vi "PMR_Main.vi"() -> ()   [LabVIEW 2016, in "Budda_V2.lvrbt"]
uses:
  Budda_V2.lvrbt
  <vilib>/NXT/Block Support/NXT_InputPort.ctl
  <vilib>/NXT/Subs/ColorSensorColors.ctl
  <vilib>/NXT/Block Support/NXT_OutputPort.ctl
  <vilib>/NXT/Dual Mode Library/Sensors/EV3_Color_Color.vi
  <vilib>/NXT/Dual Mode Library/Sensors/EV3_Ultrasonic_CM.vi
  <vilib>/NXT/NXTIO Xnodes/NXTIONodeSubVIs/NXTMoveMotors.vi
  <vilib>/NXT/Dual Mode Library/Sensors/EV3_Gyro_Reset.vi
  <vilib>/NXT/Dual Mode Library/Sensors/EV3_Gyro_Angle.vi
  <vilib>/NXT/NXTIO Xnodes/NXTIONodeSubVIs/NXTStopMotors.vi
  <vilib>/NXT/Dual Mode Library/Sensors/EV3_Gyro_Rate.vi
  <vilib>/NXT/Dual Mode Library/Sound/PlayC.vi
  <vilib>/NXT/Dual Mode Library/Sound/PlayG.vi
  <vilib>/NXT/Subs/LVHSConnector.ctl
  <vilib>/NXT/NXTIO Xnodes/AddressXNode/NXTIOAddress.xnode
  <vilib>/NXT/NXTIO Xnodes/NXTIOXNode/NXTIO.xnode
  <vilib>/NXT/LegoClasses/BrickReference/BrickReference.lvclass
panel:
  in  "Nav Speed":dbl=40.0
  in  "-Grab Power":dbl=-50.0
  in  "-Turn Speed":dbl=-45.0
  out "Drop Counter":dbl
  out "Weight":string
  out "Ultrasonic Distance":dbl
  out "Current State":string
  in  "UTurn Time":dbl=2400.0
  in  "Grab Power":dbl=80.0
  in  "Weight Threshold":dbl=-20.0
  in  "Pickup Distance":dbl=7.0
  in  "Turn speed":dbl=45.0
  in  "Drive Speed":dbl=40.0
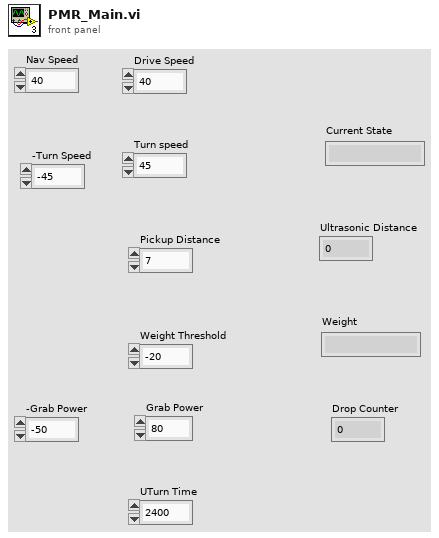
[diagram p1: front panel]
types:
  T1 = typedef "ColorSensorColors.ctl" = enum16{"No Color", "Black", "Blue", "Green", "Yellow", "Red", "White", "Brown"}
  T2 = typedef "NXT_InputPort.ctl" = u32
  T3 = typedef "NXT_OutputPort.ctl" = u8
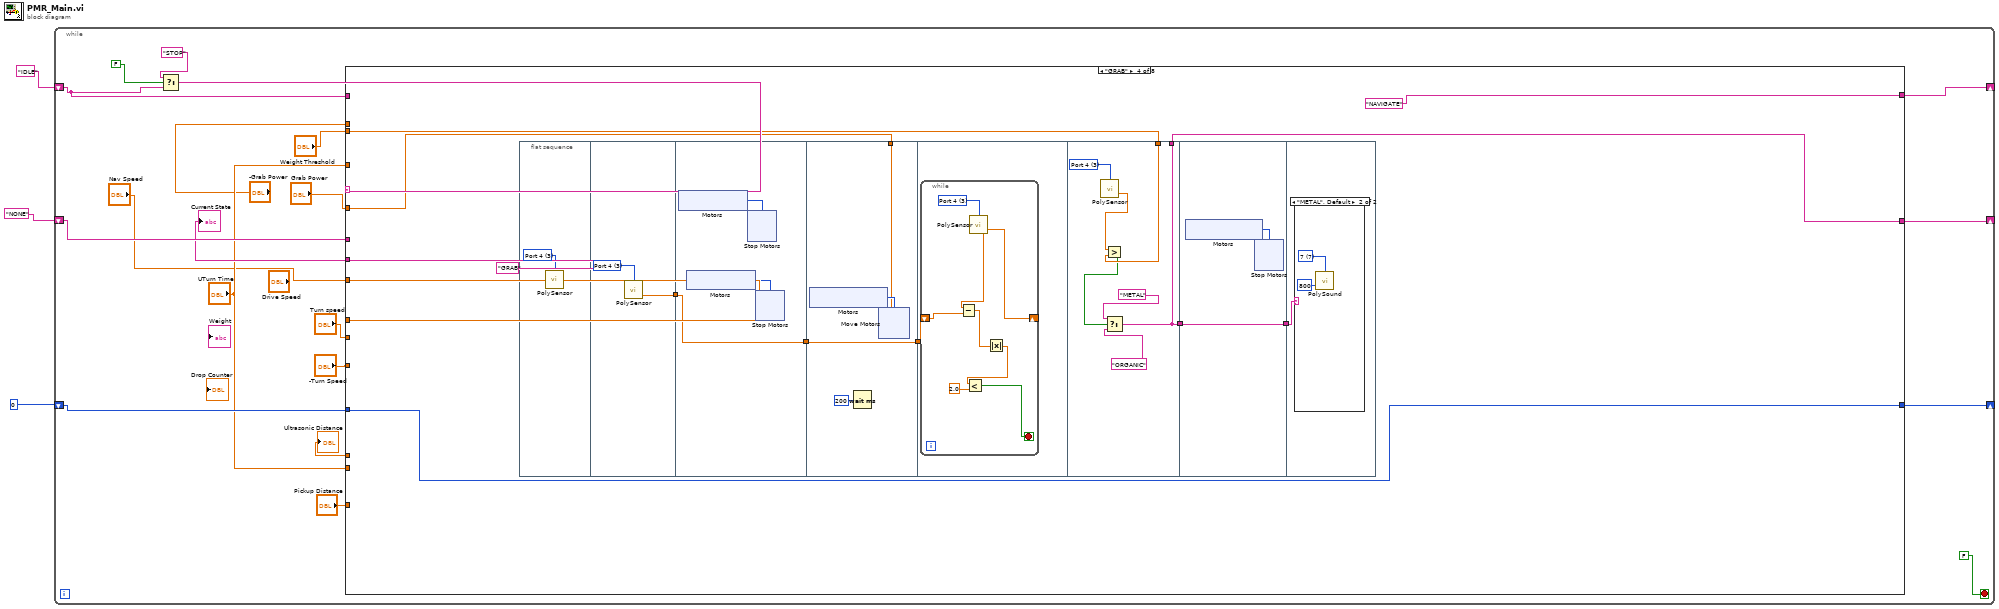
[diagram p0: block diagram]
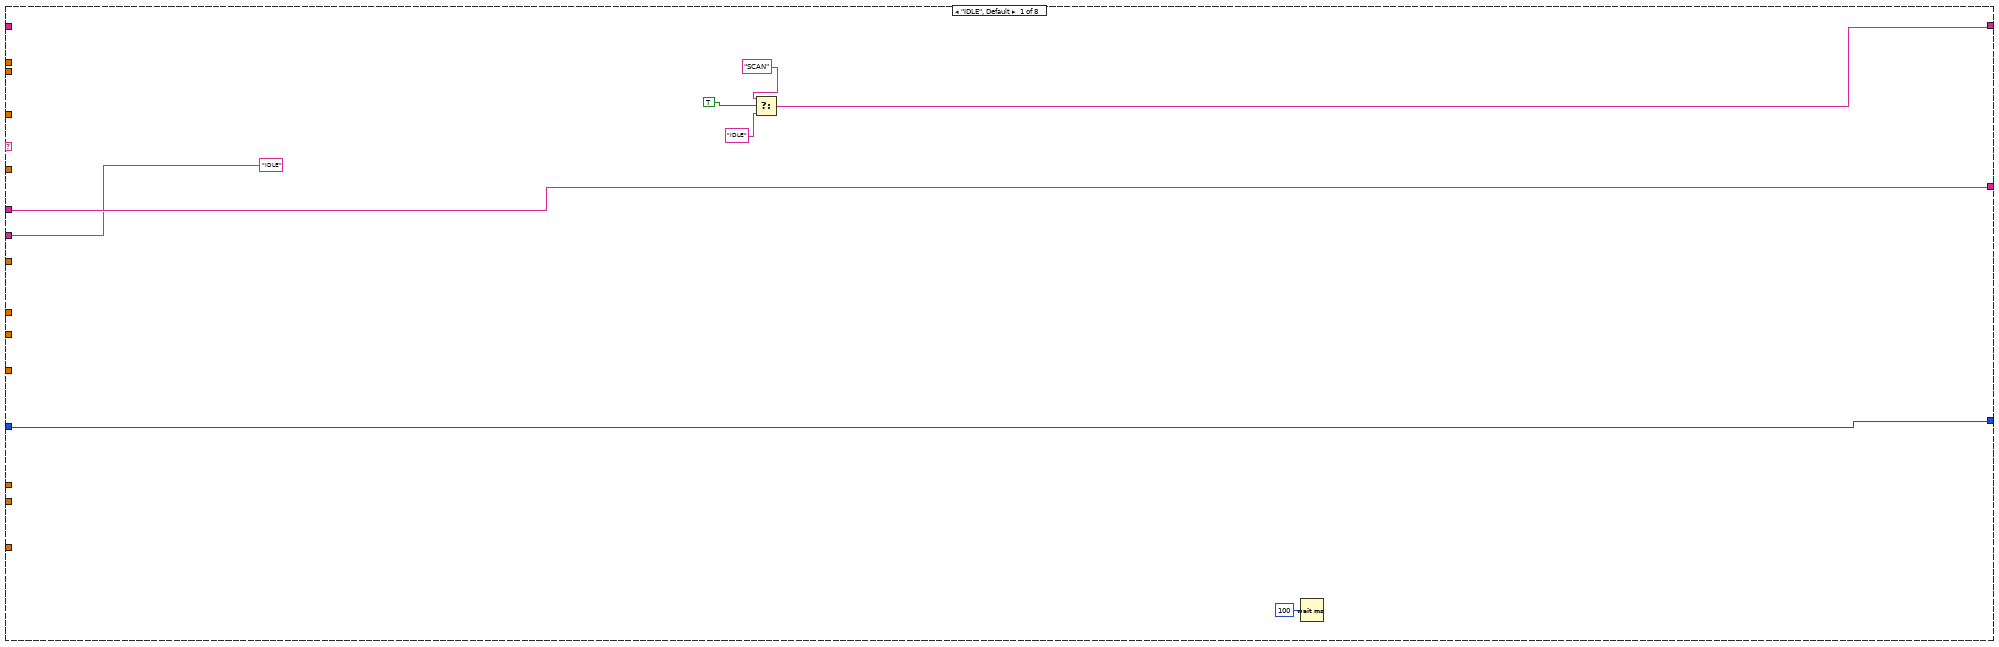
[diagram p2: hidden frame]
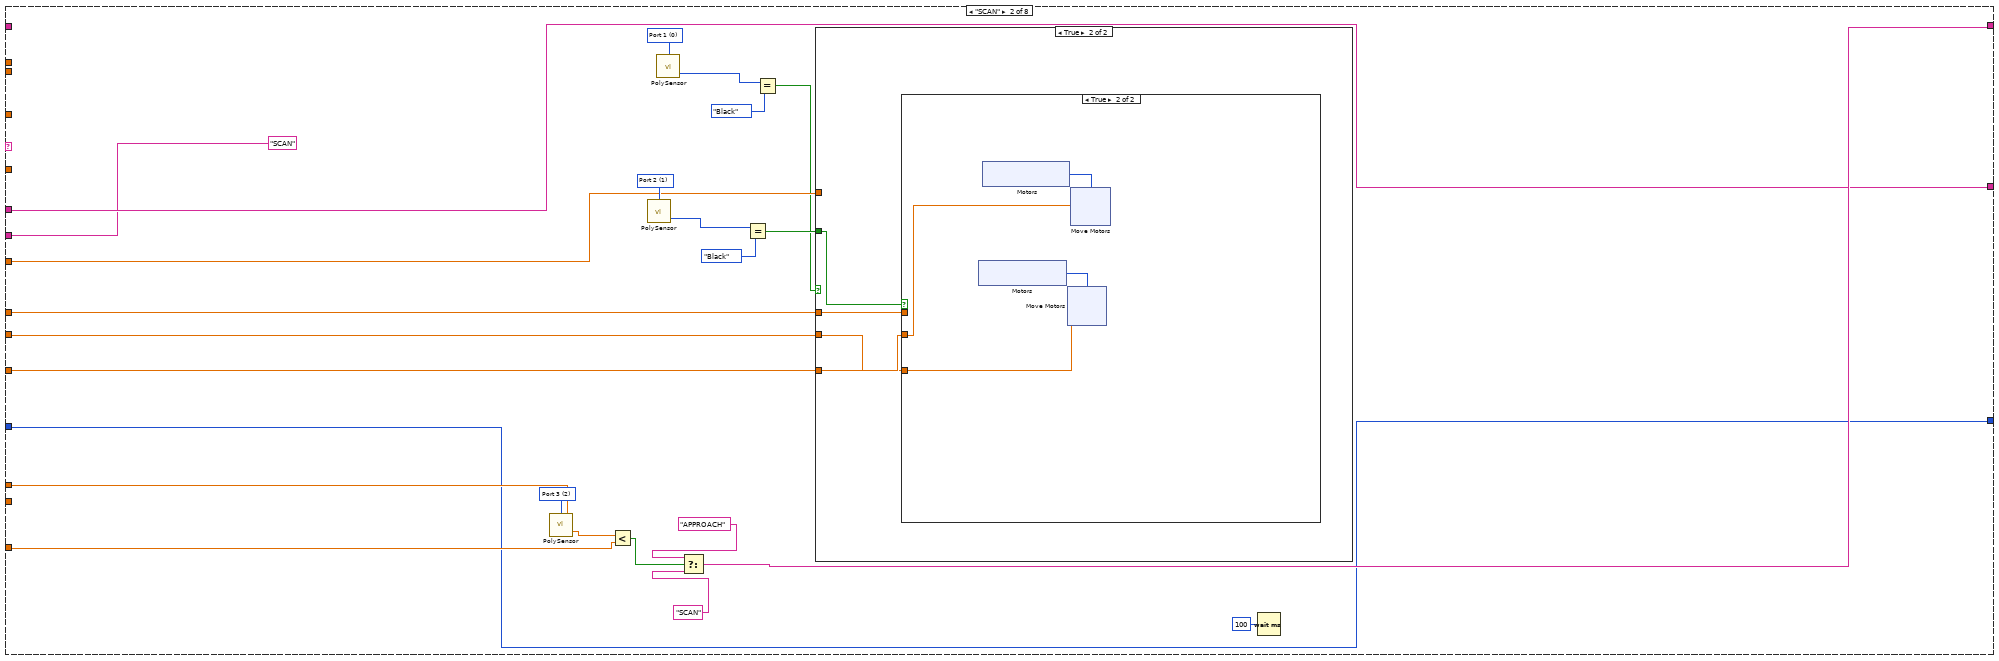
[diagram p3: hidden frame]
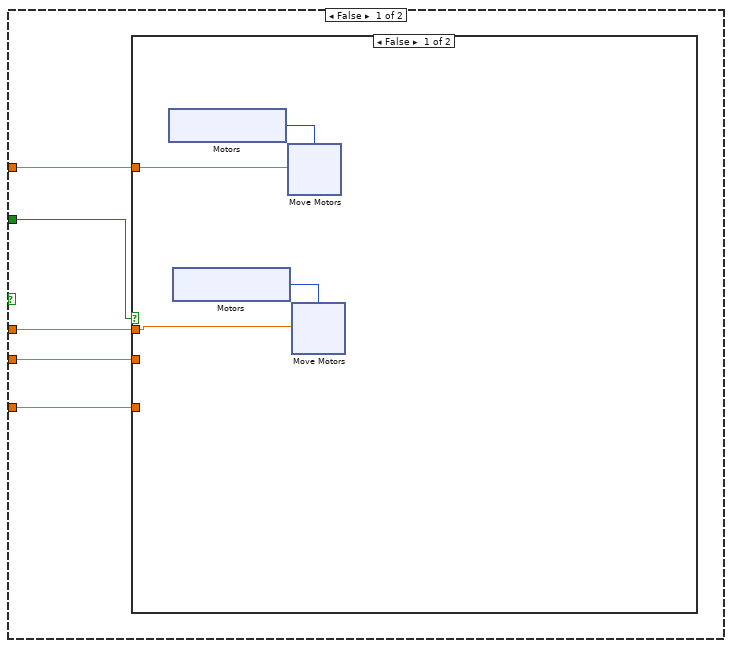
[diagram p4: hidden frame]
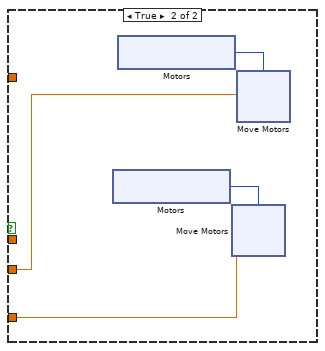
[diagram p5: hidden frame]
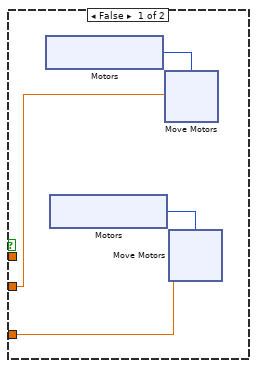
[diagram p6: hidden frame]
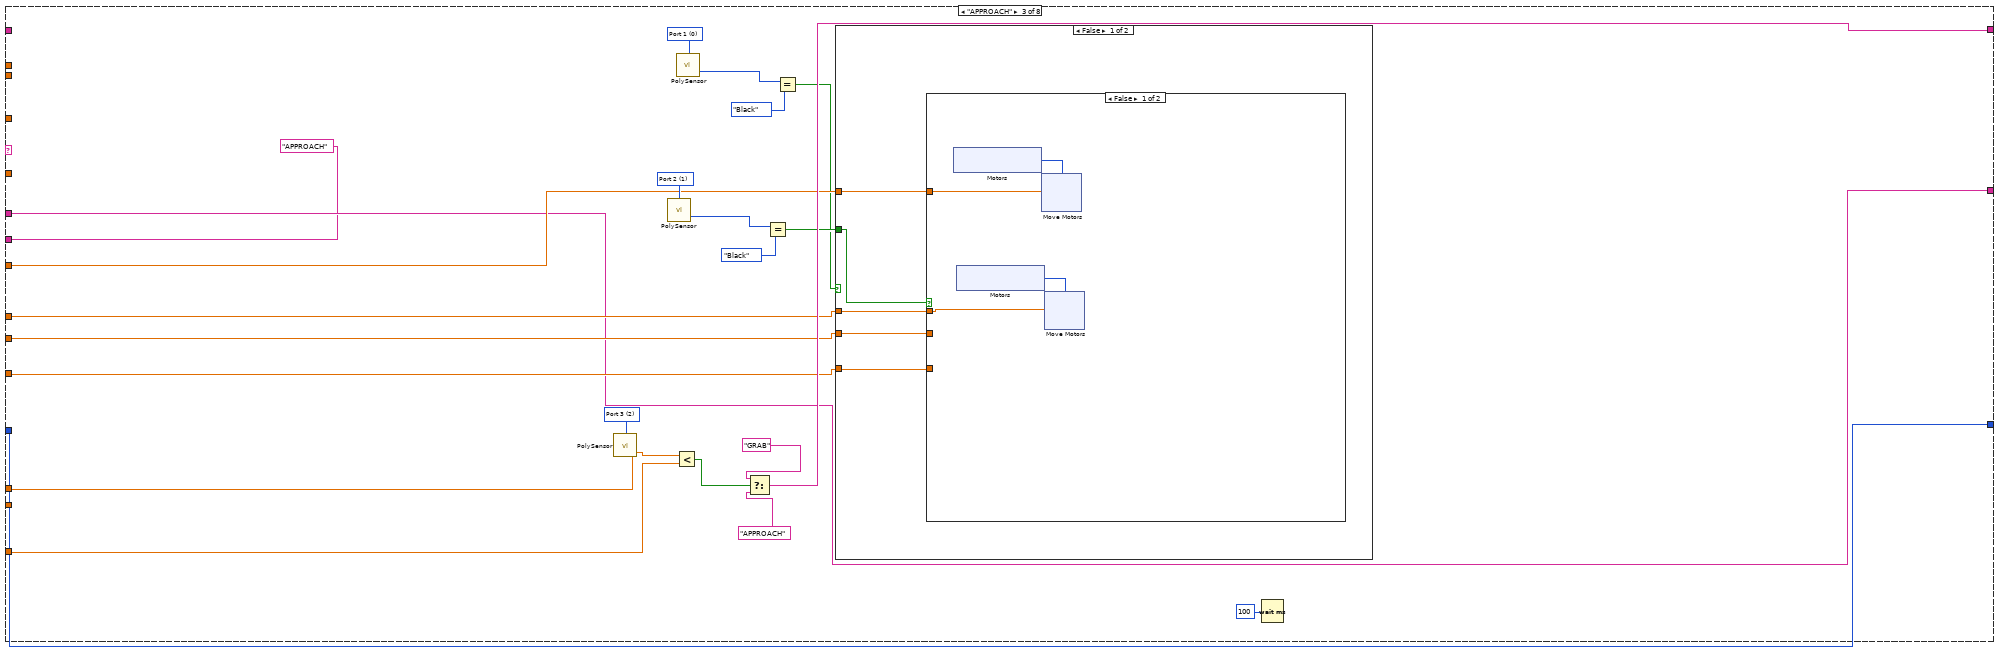
[diagram p7: hidden frame]
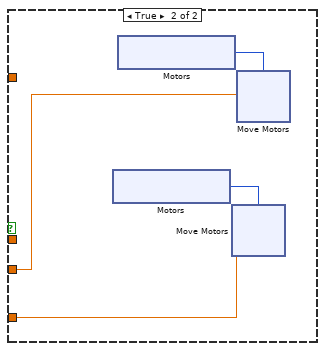
[diagram p8: hidden frame]
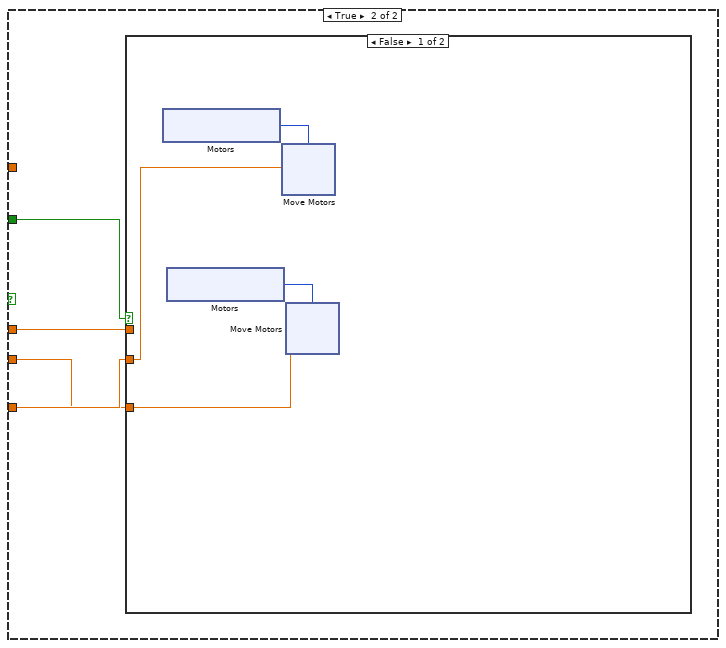
[diagram p9: hidden frame]
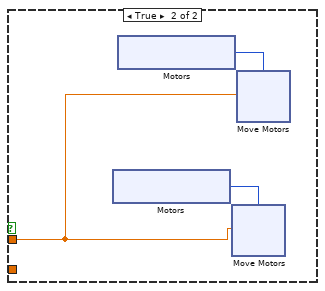
[diagram p10: hidden frame]
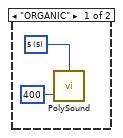
[diagram p11: hidden frame]
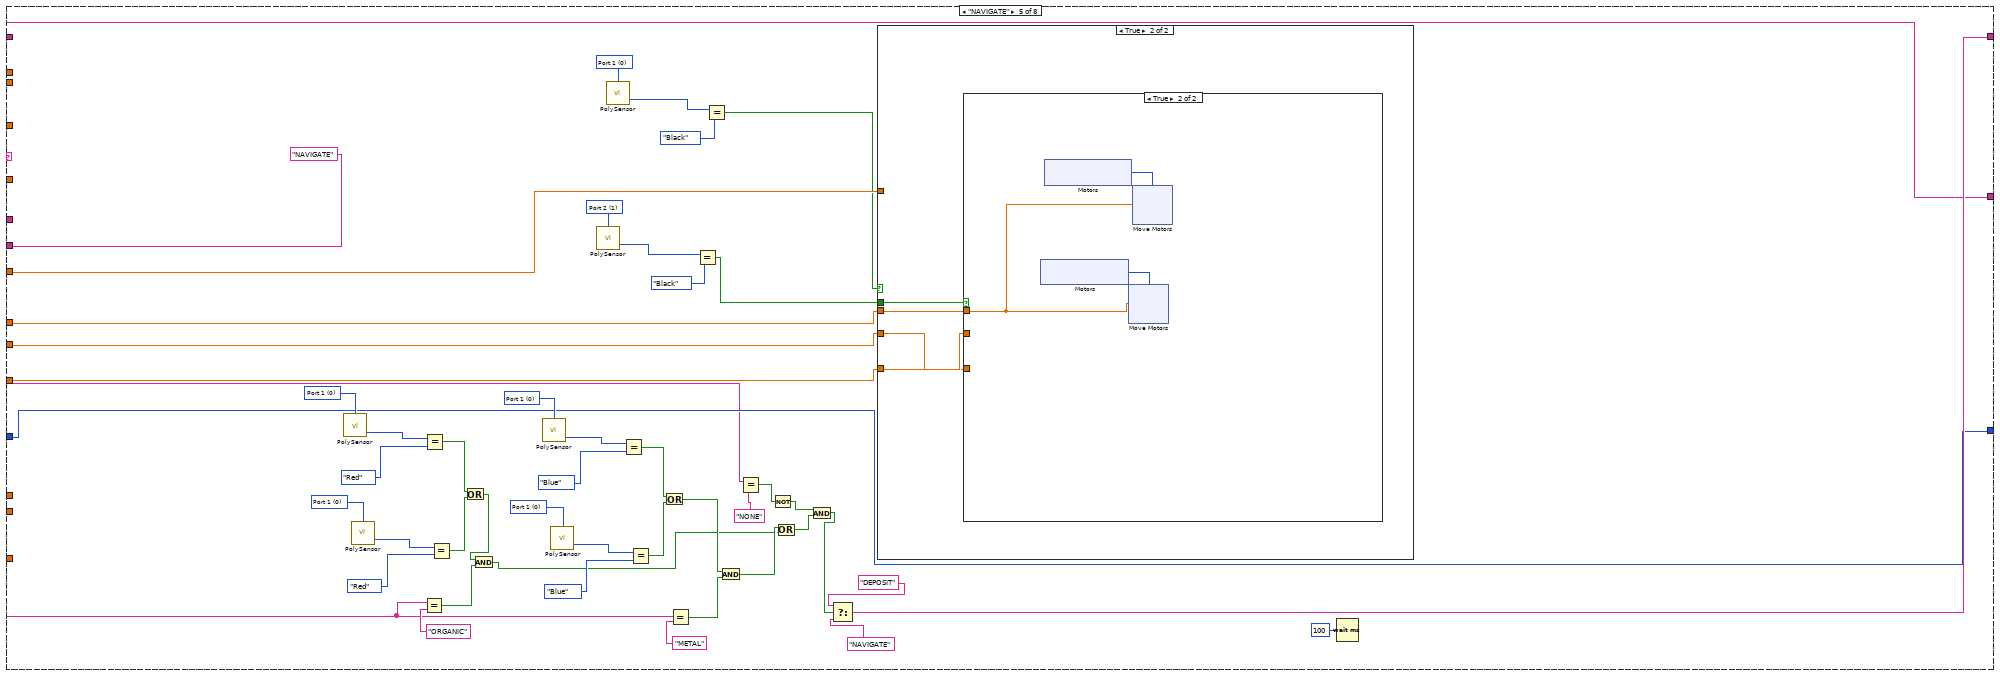
[diagram p12: hidden frame]
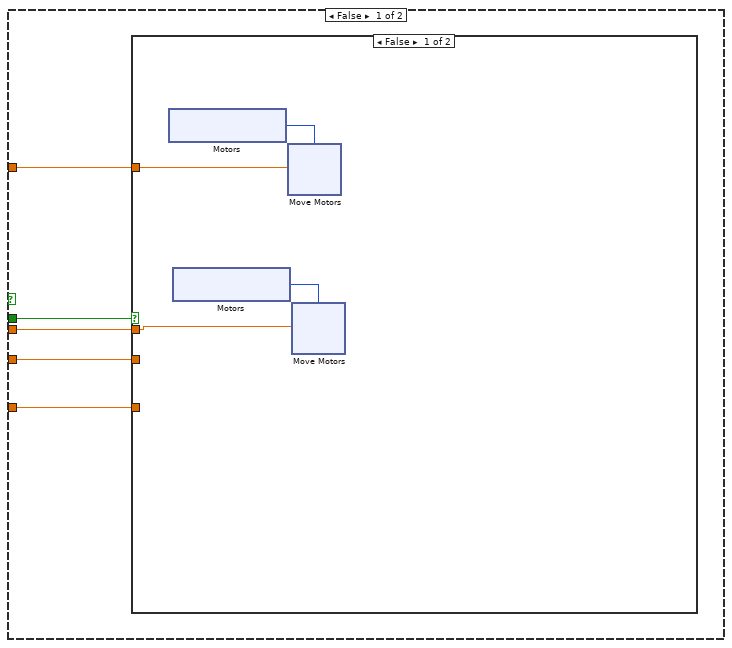
[diagram p13: hidden frame]
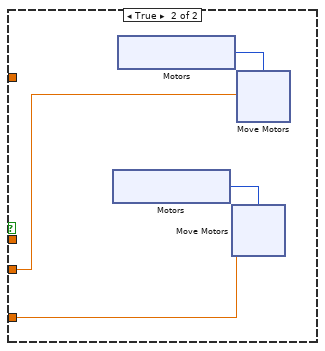
[diagram p14: hidden frame]
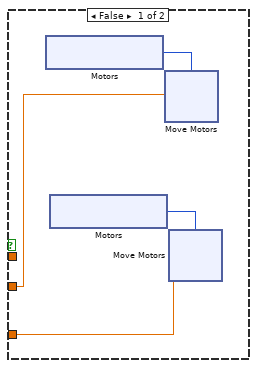
[diagram p15: hidden frame]
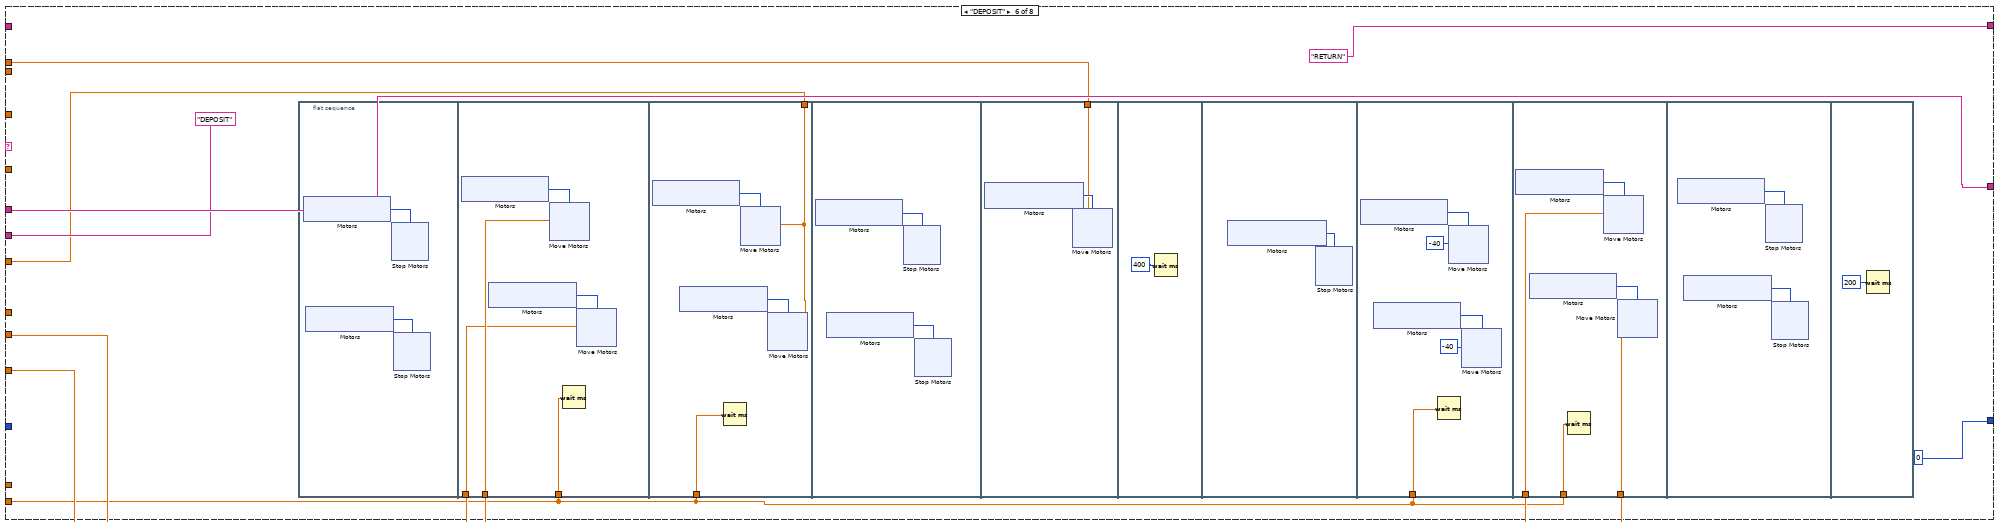
[diagram p16: hidden frame]
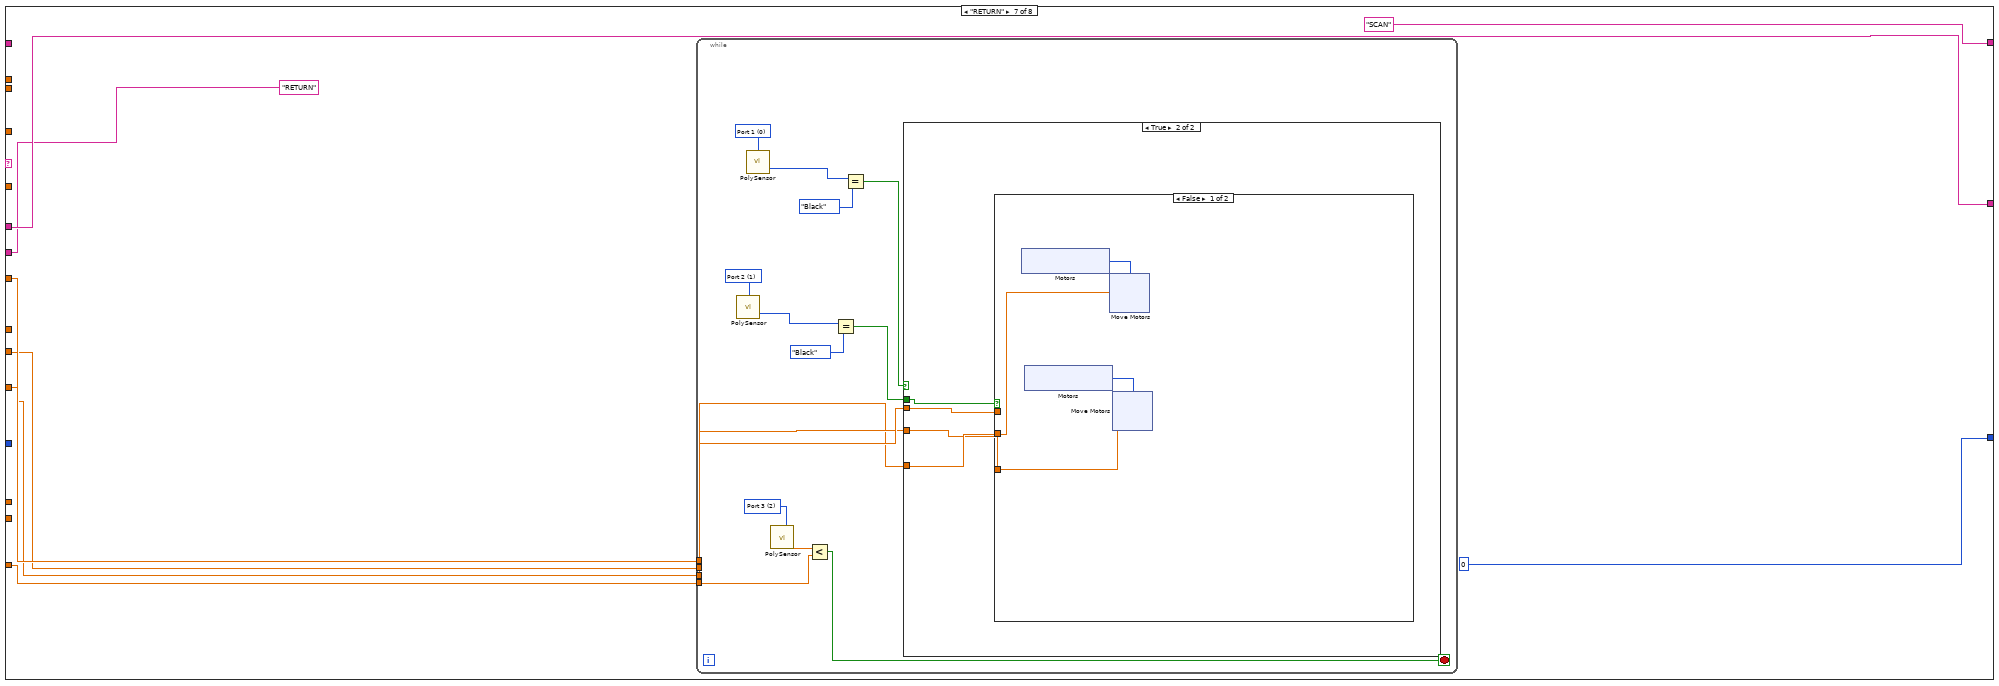
[diagram p17: hidden frame]
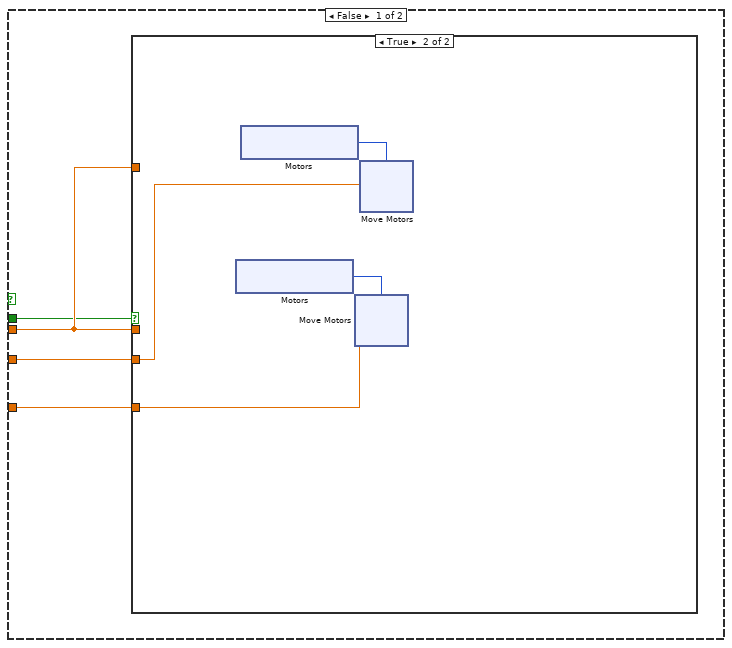
[diagram p18: hidden frame]
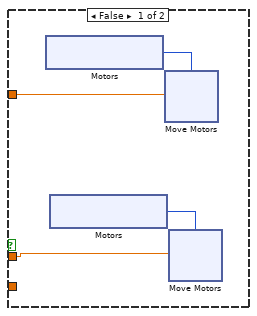
[diagram p19: hidden frame]
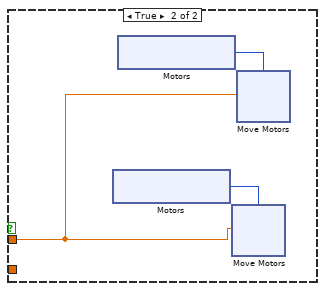
[diagram p20: hidden frame]
diagram:
  n1 = while {
    shift-right: [w11] -> _
    shift-left: "IDLE" -> [w21]
    shift-right: [w10] -> _
    shift-left: "NONE" -> [w20]
    shift-right: [w9] -> _
    shift-left: 0 -> [w19]
    stop <- FALSE stop-if-true
    n2 = Select(t="STOP", s=FALSE, f=w21) -> (s? t:f=w22:string)
    n3 = case shown="\"GRAB\"" w22 {
      tunnel: [w28 w38 w154 "NAVIGATE" w331 "RETURN" "SCAN" "IDLE"] -> w11
      tunnel: w21 -> [_ _ _ _ _ _ _ _]
      tunnel: [w26 w37 w149 w263 w327 w466 w616 w724] -> w10
      tunnel: w20 -> [w26 w37 w149 _ w327 w466 w616 w724]
      tunnel: [w31 w36 w148 w261 w330 0 0 0] -> w9
      tunnel: w19 -> [w31 w36 w148 w261 w330 _ _ _]
      tunnel: "Nav Speed" -> [_ w48 w150 _ w362 w464 w620 _]
      tunnel: "Nav Speed" -> [_ w47 w153 _ w365 _ _ _]
      tunnel: "Turn speed" -> [_ w46 w152 _ w364 w462 w613 _]
      tunnel: "-Turn Speed" -> [_ w45 w151 _ w363 w461 w614 _]
      tunnel: [_ w43 w155 _ _ _ _ _] -> w16
      tunnel: "Pickup Distance" -> [_ w42 w156 _ _ _ w619 _]
      tunnel: "Grab Power" -> [_ _ _ w265 _ _ _ _]
      tunnel: "Weight Threshold" -> [_ _ _ w264 _ _ _ _]
      tunnel: ["IDLE" "SCAN" "APPROACH" "GRAB" "NAVIGATE" "DEPOSIT" "RETURN" "STOP"] -> w12
      tunnel: "UTurn Time" -> [_ _ _ _ _ _ _ _]
      tunnel: "UTurn Time" -> [_ _ _ _ _ w460 _ _]
      tunnel: "-Grab Power" -> [_ _ _ _ _ w463 _ _]
      frame "IDLE", Default {
        n4 = Select(t="SCAN", s=TRUE, f="IDLE") -> (s? t:f=w28:string)
        n5 = Wait (ms)(milliseconds to wait=u32 100) -> ()  [unwired: 1 out]
      }
      frame "SCAN" {
        w44 = T2 2 items=["Port 1", "Port 2", "Port 3", "Port 4"] ("Port (Port 1)")
        w51 = T2 1 items=["Port 1", "Port 2", "Port 3", "Port 4"] ("Port (Port 1)")
        w54 = T2 0 items=["Port 1", "Port 2", "Port 3", "Port 4"] ("Port (Port 1)")
        n6 = call-poly <vilib>:"PolySensor.vi"("Port (Port 1)"=w44) -> ("Centimeters"=w43:sgl)  [unwired: 2 in, 1 out]
        n7 = Less?(x=w43, y=w42) -> (x < y?=w41:bool)
        n8 = call-poly <vilib>:"PolySensor.vi"("Port (Port 1)"=w51) -> ("Detected Color"=w50:T1)  [unwired: 2 in, 1 out]
        n9 = call-poly <vilib>:"PolySensor.vi"("Port (Port 1)"=w54) -> ("Detected Color"=w53:T1)  [unwired: 2 in, 1 out]
        n10 = Select(t="APPROACH", s=w41, f="SCAN") -> (s? t:f=w38:string)
        n11 = Equal?(x=w50, y=ColorSensorColors."Black") -> (x = y?=w33:bool)
        n12 = Equal?(x=w53, y=ColorSensorColors."Black") -> (x = y?=w32:bool)
        n13 = case shown="True" w32 {
          tunnel: w48 -> [w59 _]
          tunnel: w47 -> [w58 w101]
          tunnel: w46 -> [w57 w102]
          tunnel: w45 -> [w56 w103]
          tunnel: w33 -> [w55 w100]
          frame False {
            n14 = case shown="False" w55 {
              tunnel: w59 -> [w61 _]
              tunnel: w58 -> [w60 _]
              tunnel: w57 -> [_ w81]
              tunnel: w56 -> [_ w80]
              frame False {
                n15 = xnode "Motors"() -> ("Motor"=w63:T3)
                n16 = xnode "Motors"() -> ("Motor"=w62:T3)
                n17 = xnode "Move Motors"("Power/Speed 1"=w61, "Motors"=w63) -> ()  [unwired: 1 in, 1 out]
                n18 = xnode "Move Motors"("Power/Speed 1"=w60, "Motors"=w62) -> ()  [unwired: 1 in, 1 out]
              }
              frame True {
                n19 = xnode "Motors"() -> ("Motor"=w82:T3)
                n20 = xnode "Motors"() -> ("Motor"=w83:T3)
                n21 = xnode "Move Motors"("Power/Speed 1"=w80, "Motors"=w82) -> ()  [unwired: 1 in, 1 out]
                n22 = xnode "Move Motors"("Power/Speed 1"=w81, "Motors"=w83) -> ()  [unwired: 1 in, 1 out]
              }
            }
          }
          frame True {
            n23 = case shown="True" w100 {
              tunnel: w103 -> [w105 w125]
              tunnel: w102 -> [w104 w124]
              tunnel: w101 -> [_ _]
              frame False {
                n24 = xnode "Motors"() -> ("Motor"=w107:T3)
                n25 = xnode "Motors"() -> ("Motor"=w106:T3)
                n26 = xnode "Move Motors"("Power/Speed 1"=w105, "Motors"=w107) -> ()  [unwired: 1 in, 1 out]
                n27 = xnode "Move Motors"("Power/Speed 1"=w104, "Motors"=w106) -> ()  [unwired: 1 in, 1 out]
              }
              frame True {
                n28 = xnode "Motors"() -> ("Motor"=w126:T3)
                n29 = xnode "Motors"() -> ("Motor"=w127:T3)
                n30 = xnode "Move Motors"("Power/Speed 1"=w124, "Motors"=w126) -> ()  [unwired: 1 in, 1 out]
                n31 = xnode "Move Motors"("Power/Speed 1"=w125, "Motors"=w127) -> ()  [unwired: 1 in, 1 out]
              }
            }
          }
        }
        n32 = Wait (ms)(milliseconds to wait=u32 100) -> ()  [unwired: 1 out]
      }
      frame "APPROACH" {
        w160 = T2 2 items=["Port 1", "Port 2", "Port 3", "Port 4"] ("Port (Port 1)")
        w163 = T2 1 items=["Port 1", "Port 2", "Port 3", "Port 4"] ("Port (Port 1)")
        w166 = T2 0 items=["Port 1", "Port 2", "Port 3", "Port 4"] ("Port (Port 1)")
        n33 = call-poly <vilib>:"PolySensor.vi"("Port (Port 1)"=w160) -> ("Centimeters"=w155:sgl)  [unwired: 2 in, 1 out]
        n34 = call-poly <vilib>:"PolySensor.vi"("Port (Port 1)"=w163) -> ("Detected Color"=w162:T1)  [unwired: 2 in, 1 out]
        n35 = Less?(x=w155, y=w156) -> (x < y?=w159:bool)
        n36 = call-poly <vilib>:"PolySensor.vi"("Port (Port 1)"=w166) -> ("Detected Color"=w165:T1)  [unwired: 2 in, 1 out]
        n37 = Select(t="GRAB", s=w159, f="APPROACH") -> (s? t:f=w154:string)
        n38 = Equal?(x=w162, y=ColorSensorColors."Black") -> (x = y?=w145:bool)
        n39 = Equal?(x=w165, y=ColorSensorColors."Black") -> (x = y?=w144:bool)
        n40 = case shown="False" w144 {
          tunnel: w150 -> [w171 _]
          tunnel: w153 -> [w170 w213]
          tunnel: w152 -> [w169 w214]
          tunnel: w151 -> [w168 w215]
          tunnel: w145 -> [w167 w212]
          frame False {
            n41 = case shown="False" w167 {
              tunnel: w171 -> [w173 _]
              tunnel: w170 -> [w172 _]
              tunnel: w169 -> [_ w193]
              tunnel: w168 -> [_ w192]
              frame False {
                n42 = xnode "Motors"() -> ("Motor"=w175:T3)
                n43 = xnode "Motors"() -> ("Motor"=w174:T3)
                n44 = xnode "Move Motors"("Power/Speed 1"=w173, "Motors"=w175) -> ()  [unwired: 1 in, 1 out]
                n45 = xnode "Move Motors"("Power/Speed 1"=w172, "Motors"=w174) -> ()  [unwired: 1 in, 1 out]
              }
              frame True {
                n46 = xnode "Motors"() -> ("Motor"=w194:T3)
                n47 = xnode "Motors"() -> ("Motor"=w195:T3)
                n48 = xnode "Move Motors"("Power/Speed 1"=w192, "Motors"=w194) -> ()  [unwired: 1 in, 1 out]
                n49 = xnode "Move Motors"("Power/Speed 1"=w193, "Motors"=w195) -> ()  [unwired: 1 in, 1 out]
              }
            }
          }
          frame True {
            n50 = case shown="False" w212 {
              tunnel: w215 -> [w217 _]
              tunnel: w214 -> [w216 _]
              tunnel: w213 -> [_ w236]
              frame False {
                n51 = xnode "Motors"() -> ("Motor"=w219:T3)
                n52 = xnode "Motors"() -> ("Motor"=w218:T3)
                n53 = xnode "Move Motors"("Power/Speed 1"=w217, "Motors"=w219) -> ()  [unwired: 1 in, 1 out]
                n54 = xnode "Move Motors"("Power/Speed 1"=w216, "Motors"=w218) -> ()  [unwired: 1 in, 1 out]
              }
              frame True {
                n55 = xnode "Motors"() -> ("Motor"=w237:T3)
                n56 = xnode "Motors"() -> ("Motor"=w238:T3)
                n57 = xnode "Move Motors"("Power/Speed 1"=w236, "Motors"=w237) -> ()  [unwired: 1 in, 1 out]
                n58 = xnode "Move Motors"("Power/Speed 1"=w236, "Motors"=w238) -> ()  [unwired: 1 in, 1 out]
              }
            }
          }
        }
        n59 = Wait (ms)(milliseconds to wait=u32 100) -> ()  [unwired: 1 out]
      }
      frame "GRAB" {
        n60 = flat-sequence {
          tunnel: [w267] -> w257
          tunnel: w257 -> [w269]
          tunnel: [w269] -> w255
          tunnel: w265 -> [w286]
          tunnel: [w285] -> w256
          tunnel: w255 -> [w285]
          tunnel: w256 -> [w296]
          tunnel: w264 -> [w305]
          tunnel: [w308] -> w263
          tunnel: [w308] -> w258
          tunnel: [w311] -> w259
          tunnel: w258 -> [w311]
          tunnel: w259 -> [w319]
          frame #0 {
            w266 = T2 3 items=["Port 1", "Port 2", "Port 3", "Port 4"] ("Port (Port 1)")
            n61 = call-poly <vilib>:"PolySensor.vi"("Port (Port 1)"=w266) -> ()  [unwired: 3 in, 1 out]
          }
          frame #1 {
            w268 = T2 3 items=["Port 1", "Port 2", "Port 3", "Port 4"] ("Port (Port 1)")
            n62 = call-poly <vilib>:"PolySensor.vi"("Port (Port 1)"=w268) -> ("Degrees"=w267:sgl)  [unwired: 2 in, 1 out]
          }
          frame #2 {
            n63 = xnode "Motors"() -> ("Motor"=w271:T3)
            n64 = xnode "Motors"() -> ("Motor"=w270:T3)
            n65 = xnode "Stop Motors"("Motors"=w271) -> ()  [unwired: 1 in, 1 out]
            n66 = xnode "Stop Motors"("Motors"=w270) -> ()  [unwired: 1 in, 1 out]
          }
          frame #3 {
            n67 = xnode "Motors"() -> ("Motor"=w287:T3)
            n68 = Wait (ms)(milliseconds to wait=u32 200) -> ()  [unwired: 1 out]
            n69 = xnode "Move Motors"("Power/Speed 1"=w286, "Motors"=w287) -> ()  [unwired: 1 in, 1 out]
          }
          frame #4 {
            n70 = while {
              shift-right: [w297] -> _
              shift-left: w296 -> [w298]
              stop <- w299 stop-if-true
              w303 = T2 3 items=["Port 1", "Port 2", "Port 3", "Port 4"] ("Port (Port 1)")
              n71 = call-poly <vilib>:"PolySensor.vi"("Port (Port 1)"=w303) -> ("Degrees"=w297:sgl)  [unwired: 2 in, 1 out]
              n72 = Subtract(x=w297, y=w298) -> (x-y=w302:sgl)
              n73 = Absolute Value(x=w302) -> (abs(x)=w301:sgl)
              n74 = Less?(x=w301, y=sgl 2.0) -> (x < y?=w299:bool)
            }
          }
          frame #5 {
            w307 = T2 3 items=["Port 1", "Port 2", "Port 3", "Port 4"] ("Port (Port 1)")
            n75 = call-poly <vilib>:"PolySensor.vi"("Port (Port 1)"=w307) -> ("Degrees/Second"=w306:sgl)  [unwired: 2 in, 1 out]
            n76 = Greater?(x=w306, y=w305) -> (0:w304:bool)
            n77 = Select(t="METAL", s=w304, f="ORGANIC") -> (s? t:f=w308:string)
          }
          frame #6 {
            n78 = xnode "Motors"() -> ("Motor"=w312:T3)
            n79 = xnode "Stop Motors"("Motors"=w312) -> ()  [unwired: 1 in, 1 out]
          }
          frame #7 {
            n80 = case shown="\"METAL\", Default" w319 {
              frame "ORGANIC" {
                w320 = u16 5 items=["3"=3, "4"=4, "5"=5, "6"=6, "7"=7] ("Octave")
                n81 = call-poly <vilib>:"PolySound.vi"("Duration (500 ms)"=u16 400, "Octave"=w320) -> ()  [unwired: 2 in, 1 out]
              }
              frame "METAL", Default {
                w322 = u16 7 items=["3"=3, "4"=4, "5"=5, "6"=6, "7"=7] ("Octave")
                n82 = call-poly <vilib>:"PolySound.vi"("Duration (500 ms)"=u16 800, "Octave"=w322) -> ()  [unwired: 2 in, 1 out]
              }
            }
          }
        }
      }
      frame "NAVIGATE" {
        w346 = T2 0 items=["Port 1", "Port 2", "Port 3", "Port 4"] ("Port (Port 1)")
        w349 = T2 0 items=["Port 1", "Port 2", "Port 3", "Port 4"] ("Port (Port 1)")
        w354 = T2 0 items=["Port 1", "Port 2", "Port 3", "Port 4"] ("Port (Port 1)")
        w357 = T2 0 items=["Port 1", "Port 2", "Port 3", "Port 4"] ("Port (Port 1)")
        w368 = T2 1 items=["Port 1", "Port 2", "Port 3", "Port 4"] ("Port (Port 1)")
        w371 = T2 0 items=["Port 1", "Port 2", "Port 3", "Port 4"] ("Port (Port 1)")
        n83 = call-poly <vilib>:"PolySensor.vi"("Port (Port 1)"=w357) -> ("Detected Color"=w356:T1)  [unwired: 2 in, 1 out]
        n84 = call-poly <vilib>:"PolySensor.vi"("Port (Port 1)"=w354) -> ("Detected Color"=w353:T1)  [unwired: 2 in, 1 out]
        n85 = Equal?(x=w327, y="ORGANIC") -> (x = y?=w337:bool)
        n86 = Equal?(x=w356, y=ColorSensorColors."Red" ("Detected Color")) -> (x = y?=w351:bool)
        n87 = Equal?(x=w353, y=ColorSensorColors."Red" ("Detected Color")) -> (x = y?=w350:bool)
        n88 = Or(x=w351, y=w350) -> (x .or. y?=w336:bool)
        n89 = And(x=w336, y=w337) -> (x .and. y?=w334:bool)
        n90 = call-poly <vilib>:"PolySensor.vi"("Port (Port 1)"=w349) -> ("Detected Color"=w348:T1)  [unwired: 2 in, 1 out]
        n91 = call-poly <vilib>:"PolySensor.vi"("Port (Port 1)"=w346) -> ("Detected Color"=w345:T1)  [unwired: 2 in, 1 out]
        n92 = call-poly <vilib>:"PolySensor.vi"("Port (Port 1)"=w368) -> ("Detected Color"=w367:T1)  [unwired: 2 in, 1 out]
        n93 = call-poly <vilib>:"PolySensor.vi"("Port (Port 1)"=w371) -> ("Detected Color"=w370:T1)  [unwired: 2 in, 1 out]
        n94 = Equal?(x=w348, y=ColorSensorColors."Blue" ("Detected Color")) -> (x = y?=w343:bool)
        n95 = Equal?(x=w345, y=ColorSensorColors."Blue" ("Detected Color")) -> (x = y?=w342:bool)
        n96 = Or(x=w343, y=w342) -> (x .or. y?=w341:bool)
        n97 = Equal?(x=w327, y="METAL") -> (x = y?=w339:bool)
        n98 = Equal?(x=w367, y=ColorSensorColors."Black") -> (x = y?=w358:bool)
        n99 = Equal?(x=w370, y=ColorSensorColors."Black") -> (x = y?=w359:bool)
        n100 = And(x=w341, y=w339) -> (x .and. y?=w335:bool)
        n101 = Equal?(x=w327, y="NONE") -> (x = y?=w329:bool)
        n102 = Not(x=w329) -> (.not. x?=w326:bool)
        n103 = Or(x=w335, y=w334) -> (x .or. y?=w325:bool)
        n104 = And(x=w326, y=w325) -> (x .and. y?=w324:bool)
        n105 = Select(t="DEPOSIT", s=w324, f="NAVIGATE") -> (s? t:f=w331:string)
        n106 = case shown="True" w359 {
          tunnel: w362 -> [w376 _]
          tunnel: w365 -> [w375 w418]
          tunnel: w364 -> [w374 w419]
          tunnel: w363 -> [w373 w420]
          tunnel: w358 -> [w372 w417]
          frame False {
            n107 = case shown="False" w372 {
              tunnel: w376 -> [w378 _]
              tunnel: w375 -> [w377 _]
              tunnel: w374 -> [_ w398]
              tunnel: w373 -> [_ w397]
              frame False {
                n108 = xnode "Motors"() -> ("Motor"=w380:T3)
                n109 = xnode "Motors"() -> ("Motor"=w379:T3)
                n110 = xnode "Move Motors"("Power/Speed 1"=w378, "Motors"=w380) -> ()  [unwired: 1 in, 1 out]
                n111 = xnode "Move Motors"("Power/Speed 1"=w377, "Motors"=w379) -> ()  [unwired: 1 in, 1 out]
              }
              frame True {
                n112 = xnode "Motors"() -> ("Motor"=w399:T3)
                n113 = xnode "Motors"() -> ("Motor"=w400:T3)
                n114 = xnode "Move Motors"("Power/Speed 1"=w397, "Motors"=w399) -> ()  [unwired: 1 in, 1 out]
                n115 = xnode "Move Motors"("Power/Speed 1"=w398, "Motors"=w400) -> ()  [unwired: 1 in, 1 out]
              }
            }
          }
          frame True {
            n116 = case shown="True" w417 {
              tunnel: w420 -> [w422 _]
              tunnel: w419 -> [w421 _]
              tunnel: w418 -> [_ w441]
              frame False {
                n117 = xnode "Motors"() -> ("Motor"=w424:T3)
                n118 = xnode "Motors"() -> ("Motor"=w423:T3)
                n119 = xnode "Move Motors"("Power/Speed 1"=w422, "Motors"=w424) -> ()  [unwired: 1 in, 1 out]
                n120 = xnode "Move Motors"("Power/Speed 1"=w421, "Motors"=w423) -> ()  [unwired: 1 in, 1 out]
              }
              frame True {
                n121 = xnode "Motors"() -> ("Motor"=w442:T3)
                n122 = xnode "Motors"() -> ("Motor"=w443:T3)
                n123 = xnode "Move Motors"("Power/Speed 1"=w441, "Motors"=w442) -> ()  [unwired: 1 in, 1 out]
                n124 = xnode "Move Motors"("Power/Speed 1"=w441, "Motors"=w443) -> ()  [unwired: 1 in, 1 out]
              }
            }
          }
        }
        n125 = Wait (ms)(milliseconds to wait=u32 100) -> ()  [unwired: 1 out]
      }
      frame "DEPOSIT" {
        n126 = flat-sequence {
          tunnel: w460 -> [w485]
          tunnel: w461 -> [w484]
          tunnel: w462 -> [w483]
          tunnel: w464 -> [w505]
          tunnel: w460 -> [w504]
          tunnel: w463 -> [w538]
          tunnel: w460 -> [w556]
          tunnel: w462 -> [w579]
          tunnel: w461 -> [w578]
          tunnel: w460 -> [w577]
          frame #0 {
            n127 = xnode "Motors"() -> ("Motor"=w469:T3)
            n128 = xnode "Motors"() -> ("Motor"=w470:T3)
            n129 = xnode "Stop Motors"("Motors"=w469) -> ()  [unwired: 1 in, 1 out]
            n130 = xnode "Stop Motors"("Motors"=w470) -> ()  [unwired: 1 in, 1 out]
          }
          frame #1 {
            n131 = xnode "Motors"() -> ("Motor"=w487:T3)
            n132 = xnode "Motors"() -> ("Motor"=w486:T3)
            n133 = xnode "Move Motors"("Power/Speed 1"=w484, "Motors"=w487) -> ()  [unwired: 1 in, 1 out]
            n134 = Wait (ms)(milliseconds to wait=w485) -> ()  [unwired: 1 out]
            n135 = xnode "Move Motors"("Power/Speed 1"=w483, "Motors"=w486) -> ()  [unwired: 1 in, 1 out]
          }
          frame #2 {
            n136 = xnode "Motors"() -> ("Motor"=w507:T3)
            n137 = xnode "Motors"() -> ("Motor"=w506:T3)
            n138 = Wait (ms)(milliseconds to wait=w504) -> ()  [unwired: 1 out]
            n139 = xnode "Move Motors"("Power/Speed 1"=w505, "Motors"=w507) -> ()  [unwired: 1 in, 1 out]
            n140 = xnode "Move Motors"("Power/Speed 1"=w505, "Motors"=w506) -> ()  [unwired: 1 in, 1 out]
          }
          frame #3 {
            n141 = xnode "Motors"() -> ("Motor"=w525:T3)
            n142 = xnode "Motors"() -> ("Motor"=w524:T3)
            n143 = xnode "Stop Motors"("Motors"=w525) -> ()  [unwired: 1 in, 1 out]
            n144 = xnode "Stop Motors"("Motors"=w524) -> ()  [unwired: 1 in, 1 out]
          }
          frame #4 {
            n145 = xnode "Motors"() -> ("Motor"=w539:T3)
            n146 = xnode "Move Motors"("Power/Speed 1"=w538, "Motors"=w539) -> ()  [unwired: 1 in, 1 out]
          }
          frame #5 {
            n147 = Wait (ms)(milliseconds to wait=u32 400) -> ()  [unwired: 1 out]
          }
          frame #6 {
            n148 = xnode "Motors"() -> ("Motor"=w549:T3)
            n149 = xnode "Stop Motors"("Motors"=w549) -> ()  [unwired: 1 in, 1 out]
          }
          frame #7 {
            n150 = xnode "Motors"() -> ("Motor"=w560:T3)
            n151 = xnode "Motors"() -> ("Motor"=w559:T3)
            n152 = Wait (ms)(milliseconds to wait=w556) -> ()  [unwired: 1 out]
            n153 = xnode "Move Motors"("Power/Speed 1"=i8 -40, "Motors"=w560) -> ()  [unwired: 1 in, 1 out]
            n154 = xnode "Move Motors"("Power/Speed 1"=i8 -40, "Motors"=w559) -> ()  [unwired: 1 in, 1 out]
          }
          frame #8 {
            n155 = xnode "Motors"() -> ("Motor"=w581:T3)
            n156 = xnode "Motors"() -> ("Motor"=w580:T3)
            n157 = Wait (ms)(milliseconds to wait=w577) -> ()  [unwired: 1 out]
            n158 = xnode "Move Motors"("Power/Speed 1"=w579, "Motors"=w581) -> ()  [unwired: 1 in, 1 out]
            n159 = xnode "Move Motors"("Power/Speed 1"=w578, "Motors"=w580) -> ()  [unwired: 1 in, 1 out]
          }
          frame #9 {
            n160 = xnode "Motors"() -> ("Motor"=w599:T3)
            n161 = xnode "Motors"() -> ("Motor"=w598:T3)
            n162 = xnode "Stop Motors"("Motors"=w599) -> ()  [unwired: 1 in, 1 out]
            n163 = xnode "Stop Motors"("Motors"=w598) -> ()  [unwired: 1 in, 1 out]
          }
          frame #10 {
            n164 = Wait (ms)(milliseconds to wait=u32 200) -> ()  [unwired: 1 out]
          }
        }
      }
      frame "RETURN" {
        n165 = while {
          tunnel: w620 -> [w629]
          tunnel: w613 -> [w628]
          tunnel: w614 -> [w627]
          tunnel: w619 -> [w624]
          stop <- w623 stop-if-true
          w626 = T2 2 items=["Port 1", "Port 2", "Port 3", "Port 4"] ("Port (Port 1)")
          w632 = T2 1 items=["Port 1", "Port 2", "Port 3", "Port 4"] ("Port (Port 1)")
          w635 = T2 0 items=["Port 1", "Port 2", "Port 3", "Port 4"] ("Port (Port 1)")
          n166 = call-poly <vilib>:"PolySensor.vi"("Port (Port 1)"=w632) -> ("Detected Color"=w631:T1)  [unwired: 2 in, 1 out]
          n167 = call-poly <vilib>:"PolySensor.vi"("Port (Port 1)"=w635) -> ("Detected Color"=w634:T1)  [unwired: 2 in, 1 out]
          n168 = call-poly <vilib>:"PolySensor.vi"("Port (Port 1)"=w626) -> ("Centimeters"=w625:sgl)  [unwired: 2 in, 1 out]
          n169 = Less?(x=w625, y=w624) -> (x < y?=w623:bool)
          n170 = Equal?(x=w631, y=ColorSensorColors."Black") -> (x = y?=w621:bool)
          n171 = Equal?(x=w634, y=ColorSensorColors."Black") -> (x = y?=w622:bool)
          n172 = case shown="True" w622 {
            tunnel: w629 -> [w637 w681]
            tunnel: w628 -> [w639 w682]
            tunnel: w627 -> [w638 w683]
            tunnel: w621 -> [w636 w680]
            frame False {
              n173 = case shown="True" w636 {
                tunnel: w637 -> [w641 _]
                tunnel: w637 -> [w640 _]
                tunnel: w639 -> [_ w661]
                tunnel: w638 -> [_ w660]
                frame False {
                  n174 = xnode "Motors"() -> ("Motor"=w643:T3)
                  n175 = xnode "Motors"() -> ("Motor"=w642:T3)
                  n176 = xnode "Move Motors"("Power/Speed 1"=w641, "Motors"=w643) -> ()  [unwired: 1 in, 1 out]
                  n177 = xnode "Move Motors"("Power/Speed 1"=w640, "Motors"=w642) -> ()  [unwired: 1 in, 1 out]
                }
                frame True {
                  n178 = xnode "Motors"() -> ("Motor"=w662:T3)
                  n179 = xnode "Motors"() -> ("Motor"=w663:T3)
                  n180 = xnode "Move Motors"("Power/Speed 1"=w660, "Motors"=w662) -> ()  [unwired: 1 in, 1 out]
                  n181 = xnode "Move Motors"("Power/Speed 1"=w661, "Motors"=w663) -> ()  [unwired: 1 in, 1 out]
                }
              }
            }
            frame True {
              n182 = case shown="False" w680 {
                tunnel: w683 -> [w685 _]
                tunnel: w682 -> [w684 _]
                tunnel: w681 -> [_ w704]
                frame False {
                  n183 = xnode "Motors"() -> ("Motor"=w687:T3)
                  n184 = xnode "Motors"() -> ("Motor"=w686:T3)
                  n185 = xnode "Move Motors"("Power/Speed 1"=w685, "Motors"=w687) -> ()  [unwired: 1 in, 1 out]
                  n186 = xnode "Move Motors"("Power/Speed 1"=w684, "Motors"=w686) -> ()  [unwired: 1 in, 1 out]
                }
                frame True {
                  n187 = xnode "Motors"() -> ("Motor"=w705:T3)
                  n188 = xnode "Motors"() -> ("Motor"=w706:T3)
                  n189 = xnode "Move Motors"("Power/Speed 1"=w704, "Motors"=w705) -> ()  [unwired: 1 in, 1 out]
                  n190 = xnode "Move Motors"("Power/Speed 1"=w704, "Motors"=w706) -> ()  [unwired: 1 in, 1 out]
                }
              }
            }
          }
        }
      }
      frame "STOP" {
        n191 = flat-sequence {
          frame #0 {
            n192 = xnode "Motors"() -> ("Motor"=w729:T3)
            n193 = xnode "Motors"() -> ("Motor"=w728:T3)
            n194 = xnode "Motors"() -> ("Motor"=w727:T3)
            n195 = xnode "Stop Motors"("Motors"=w729) -> ()  [unwired: 1 in, 1 out]
            n196 = xnode "Stop Motors"("Motors"=w728) -> ()  [unwired: 1 in, 1 out]
            n197 = xnode "Stop Motors"("Motors"=w727) -> ()  [unwired: 1 in, 1 out]
          }
          frame #1 {
            n198 = while {
              stop <- TRUE stop-if-true
              n199 = Wait (ms)(milliseconds to wait=u32 100) -> ()  [unwired: 1 out]
            }
          }
        }
      }
    }
    "Current State" <- w12
    "Ultrasonic Distance" <- w16
  }
